vi "PertPhase.vi"(8 "PertParams":dbl[](array[numeric]), 9 "PertForcing":bool, 10 "CollectedDataIn":dbl[][](array[numeric]), 11 "Time":dbl) -> (1 "CollectedDataOut":dbl[][](array[numeric]), 2 "cond":bool, 3 "outputAmp":dbl[](array[numeric]), 5 "PertForcingOut":bool)   [LabVIEW 2017]
panel:
  out "number":u32
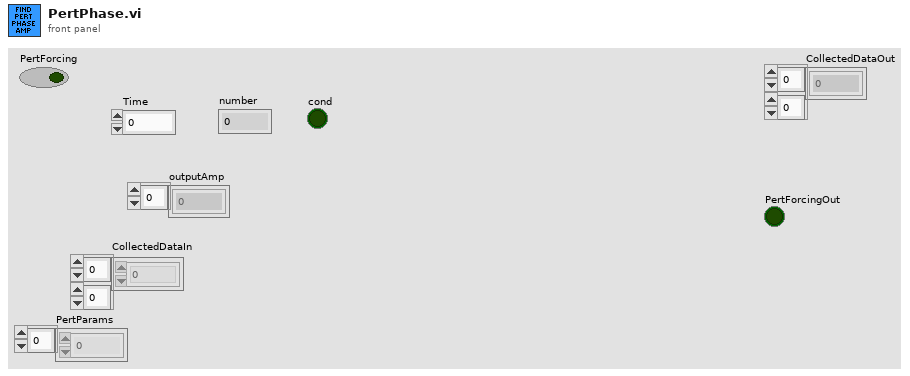
[diagram p1: front panel]
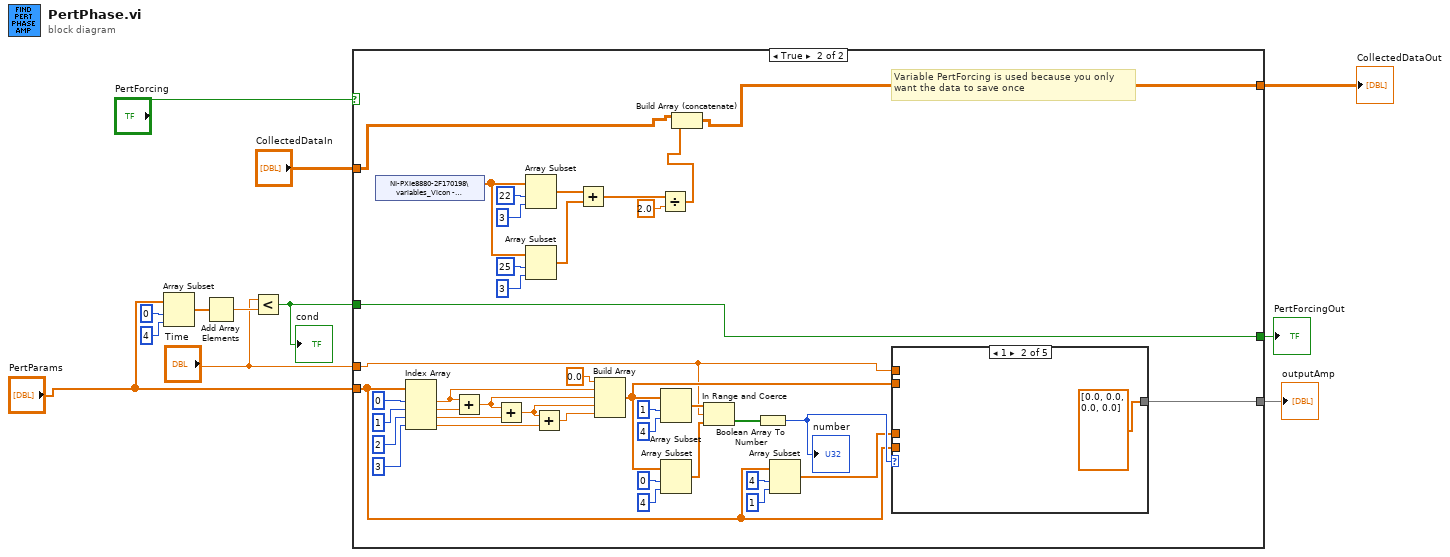
[diagram p0: block diagram]
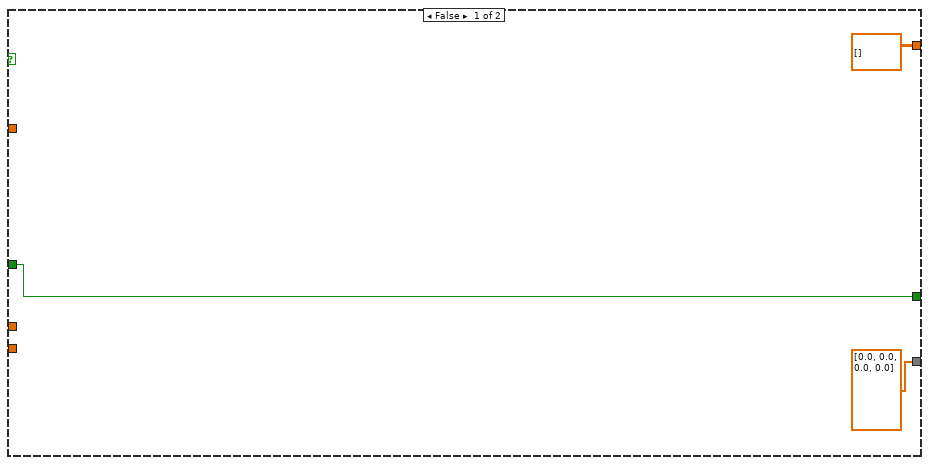
[diagram p2: hidden frame]
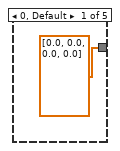
[diagram p3: hidden frame]
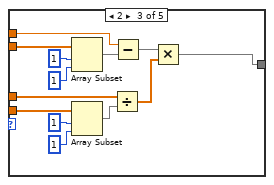
[diagram p4: hidden frame]
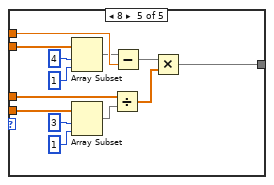
[diagram p6: hidden frame]
diagram:
  n1 = Array Subset(array="PertParams", index=0, length=4) -> (w10:dbl[])
  n2 = Add Array Elements(numeric array=w10) -> (sum=w9:dbl)
  n3 = Less?(x="Time", y=w9) -> (x < y?=w5:bool)
  "cond" <- w5
  n4 = case shown="True" "PertForcing" {
    tunnel: "PertParams" -> [_ w31]
    tunnel: "Time" -> [_ w30]
    tunnel: "CollectedDataIn" -> [_ w17]
    tunnel: [dbl[] [0.0, 0.0, 0.0, 0.0] w29] -> w7
    tunnel: [dbl[][] [] w16] -> w6
    tunnel: w5 -> [w13 w19]
    tunnel: [w13 w19] -> w2
    frame False {
    }
    frame True {
      # "Variable PertForcing is used because you only\nwant the data to save once"
      n5 = shared-variable "NI-PXIe8880-2F170198\\variables_Vicon - networkPublished.lvlib\\viconData_2"() -> (w24:dbl[])  [unwired: 1 in, 1 out]
      n6 = Index Array(array=w31, index #1=0 ("index"), index #2=1 ("index"), index #3=2 ("index"), index #4=3 ("index")) -> (element #1=w49:dbl, element #2=w48:dbl, element #3=w50:dbl, element #4=w46:dbl)
      n7 = Add(x=w49, y=w48) -> (x+y=w47:dbl)
      n8 = Add(x=w47, y=w50) -> (x+y=w38:dbl)
      n9 = Array Subset(array=w24, index=22, length=3) -> (w23:dbl[])
      n10 = Array Subset(array=w24, index=25, length=3) -> (w22:dbl[])
      n11 = Add(x=w38, y=w46) -> (x+y=w45:dbl)
      n12 = Add(x=w23, y=w22) -> (x+y=w20:dbl[])
      n13 = Build Array(0.0 ("element"), w49, w47, w38, w45) -> (w35:dbl[])
      n14 = Divide(x=w20, y=2.0) -> (x/y=w18:dbl[])
      n15 = Array Subset(array=w35, index=1, length=4) -> (w43:dbl[])
      n16 = Array Subset(array=w35, index=0, length=4) -> (w40:dbl[])
      n17 = Build Array (concatenate)(w17, w18) -> (w16:dbl[][])
      n18 = In Range and Coerce(upper limit=w43, x=w30, lower limit=w40) -> (In Range?=w37:bool[])  [unwired: 1 out]
      n19 = Boolean Array To Number(Boolean array=w37) -> (number=w36:u32)
      "number" <- w36
      n20 = Array Subset(array=w31, index=4, length=1) -> (w32:dbl[])
      n21 = case shown="1" w36 {
        tunnel: w35 -> [_ _ w70 _ w84]
        tunnel: w30 -> [_ _ w67 _ w81]
        tunnel: w32 -> [_ _ w61 w71 w79]
        tunnel: w31 -> [_ _ w64 _ w78]
        tunnel: [dbl[] [0.0, 0.0, 0.0, 0.0] dbl[] [0.0, 0.0, 0.0, 0.0] w58 w71 w72] -> w29
        frame 0, Default {
        }
        frame 1 {
        }
        frame 2 {
          n22 = Array Subset(array=w70, index=1, length=1) -> (w66:dbl[])
          n23 = Array Subset(array=w64, index=1, length=1) -> (w60:dbl[])
          n24 = Divide(x=w61, y=w60) -> (x/y=w59:dbl[])
          n25 = Subtract(x=w67, y=w66) -> (x-y=w65:dbl[])
          n26 = Multiply(x=w65, y=w59) -> (x*y=w58:dbl[])
        }
        frame 4 {
        }
        frame 8 {
          n27 = Array Subset(array=w84, index=4, length=1) -> (w80:dbl[])
          n28 = Array Subset(array=w78, index=3, length=1) -> (w75:dbl[])
          n29 = Divide(x=w79, y=w75) -> (x/y=w73:dbl[])
          n30 = Subtract(x=w80, y=w81) -> (x-y=w74:dbl[])
          n31 = Multiply(x=w74, y=w73) -> (x*y=w72:dbl[])
        }
      }
    }
  }
  "outputAmp" <- w7
  "CollectedDataOut" <- w6
  "PertForcingOut" <- w2
